vi "DataReadTxt.vi"(0 "Chemin Header":path, 5 "chemin Data":path, 9 "ScanlistIndex":i32, 11 "error in":errorcluster, 12 "VarParIndex":i32) -> (1 "Header String":string, 3 "VarPar":string, 4 "Data Preview":string[][](array[string]), 6 "X Array":dbl[](array[numeric]), 10 "Y Array":dbl[](array[numeric]), 13 "CurveName":string, 14 "enregistrement(s)":T1={"Entête"="", "Scan list"=[], "NbCourbe"=1, "IndCourbe"=0, "NomDon"=["RTêta;", "X&Y;"], "Session "=0, "Date"="", "Time"="", "VarParams"=[], "UserName"="", "ScanTableSize"=[], "VarPar list"=[], "DescKeyword"=""} caption="ScanParams", 15 "error out":errorcluster)   [LabVIEW 2019]
doc: "Ce VI lit les données contenu dans le fichier de sauvegarde automatique. Ces données correspondent aux valeurs prises lors du dernier balayage. La sauvegarde automatique est effectué après chaque acquisition."
uses:
  Interface Class/ScanParams.ctl
  Interface Class/ScanParamsOld.ctl
  Interface Class/Interface.lvclass
panel:
  out "AllData":dbl[][](array[numeric]) format="%#.16f"
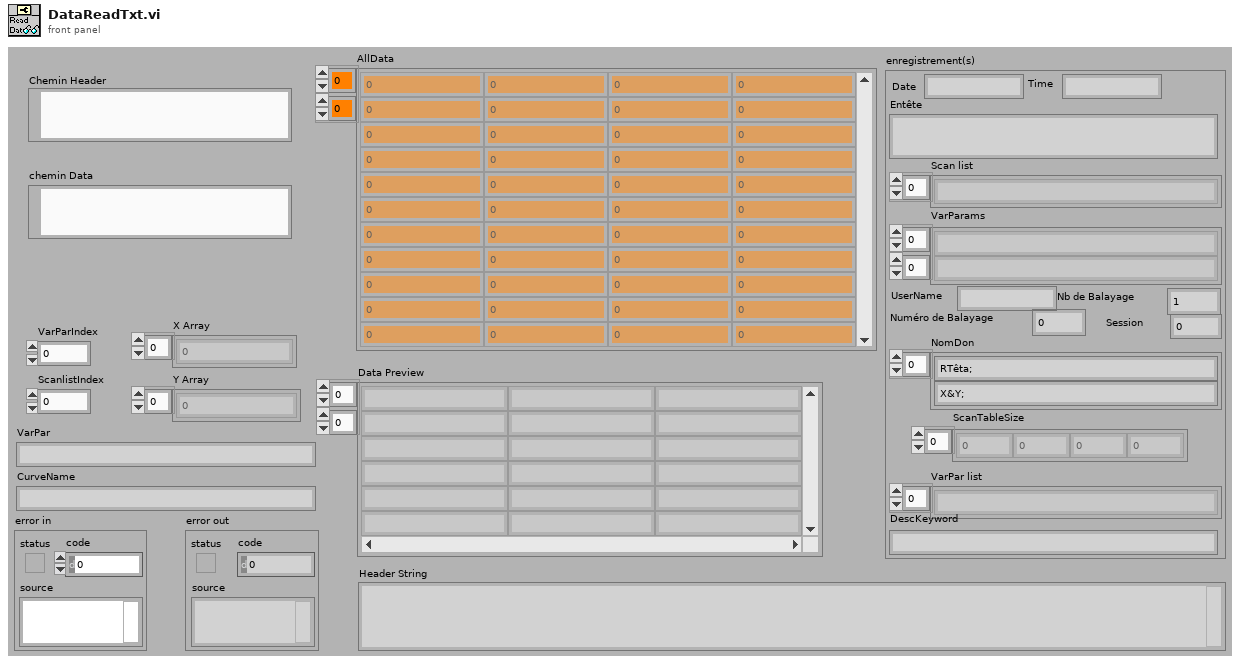
[diagram p1: front panel]
types:
  T1 = typedef "Interface.lvclass/ScanParams.ctl" = cluster{"Entête":string, "Scan list":string[], "NbCourbe":i32, "IndCourbe":i64, "NomDon":string[], "Session ":i32, "Date":string, "Time":string, "VarParams":string[][], "UserName":string, "ScanTableSize":i32[], "VarPar list":string[], "DescKeyword":string}
  T2 = typedef "Interface.lvclass/ScanParamsOld.ctl" = cluster{"Entête":string, "Scan list":string[], "NbCourbe":i32, "IndCourbe":i64, "NomDon":string[], "Session ":i32, "Date":string, "Time":string, "VarParams":string[][], "UserName":string, "ScanTableSize":i32[], "VarPar list":string[]}
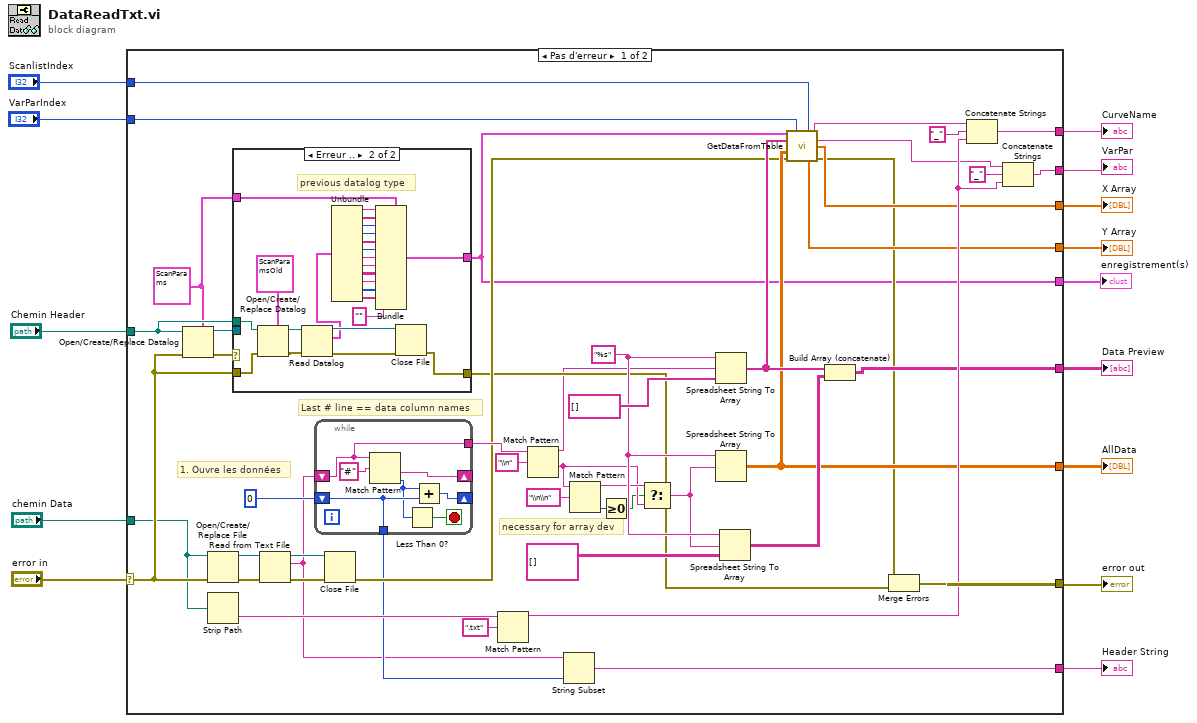
[diagram p0: block diagram]
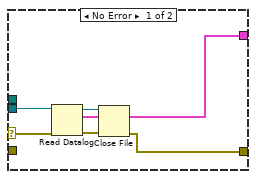
[diagram p2: hidden frame]
diagram:
  n1 = case shown="Pas d'erreur" "error in" {
    selector: "error in" -> [w31 w100]
    tunnel: "chemin Data" -> [w18 _]
    tunnel: [w33 w100] -> w14
    tunnel: [w46 _] -> w11
    tunnel: [w43 _] -> w10
    tunnel: "Chemin Header" -> [w17 _]
    tunnel: "ScanlistIndex" -> [w35 _]
    tunnel: "VarParIndex" -> [w36 _]
    tunnel: [w40 _] -> w6
    tunnel: [w39 _] -> w5
    tunnel: [w51 _] -> w4
    tunnel: [w53 _] -> w3
    tunnel: [w29 _] -> w2
    tunnel: [w15 _] -> w1
    frame No Error {
      w16 = T1 {"Entête"="", "Scan list"=[], "NbCourbe"=1, "IndCourbe"=1, "NomDon"=["RTêta;", "X&Y;"], "Session "=0, "Date"="", "Time"="", "VarParams"=[], "UserName"="", "ScanTableSize"=[], "VarPar list"=[], "DescKeyword"=""} ("ScanParams")
      w48 = "%s" ("chaîne de format")
      # "necessary for array dev"
      # "Last # line == data column names"
      # "1. Ouvre les données"
      n2 = Open/Create/Replace Datalog(5:w16, 8:w31, 11:w17) -> (0:w34:errorcluster, 3:w56:refnum<k1>)  [unwired: 3 in, 1 out]
      n3 = Open/Create/Replace File(file path (use dialog)=w18, error in=w31) -> (refnum out=w62:refnum<file>, error out=w61:errorcluster)  [unwired: 4 in, 1 out]
      n4 = Strip Path(path=w18) -> (name=w55:string)  [unwired: 1 out]
      n5 = case shown="Erreur .." w34 {
        selector: w34 -> [w65 _]
        tunnel: w56 -> [w68 _]
        tunnel: [w63 w71] -> w15
        tunnel: w17 -> [_ w87]
        tunnel: [w64 w72] -> w32
        tunnel: w31 -> [_ w70]
        tunnel: w16 -> [_ w69]
        frame No Error {
          n6 = Read Datalog(4:w65, 7:w68) -> (0:w67:errorcluster, 2:w63:T1, 3:w66:refnum<k1>)  [unwired: 1 in]
          n7 = Close File(refnum=w66, error in=w67) -> (error out=w64:errorcluster)  [unwired: 1 out]
        }
        frame Error {
          # "previous datalog type"
          n8 = Open/Create/Replace Datalog(5:T2 {"Entête"="", "Scan list"=[], "NbCourbe"=1, "IndCourbe"=1, "NomDon"=["RTêta;", "X&Y;"], "Session "=0, "Date"="", "Time"="", "VarParams"=[], "UserName"="", "ScanTableSize"=[], "VarPar list"=[]} ("ScanParams"), 8:w70, 11:w87) -> (0:w89:errorcluster, 3:w90:refnum<k1>)  [unwired: 3 in, 1 out]
          n9 = Read Datalog(4:w89, 7:w90) -> (0:w92:errorcluster, 2:w86:T2, 3:w91:refnum<k1>)  [unwired: 1 in]
          n10 = Unbundle(w86) -> ("Entête"=w85:string, "Scan list"=w84:string[], "NbCourbe"=w83:i32, "IndCourbe"=w82:i64, "NomDon"=w81:string[], "Session"=w80:i32, "Date"=w79:string, "Time"=w78:string, "VarParams"=w77:string[][], "UserName"=w76:string, "ScanTableSize"=w75:i32[], "VarPar list"=w74:string[])
          n11 = Bundle(cluster=w69, "Entête"=w85, "Scan list"=w84, "NbCourbe"=w83, "IndCourbe"=w82, "NomDon"=w81, "Session"=w80, "Date"=w79, "Time"=w78, "VarParams"=w77, "UserName"=w76, "ScanTableSize"=w75, "VarPar list"=w74, "DescKeyword"="") -> (w71:T1)
          n12 = Close File(refnum=w91, error in=w92) -> (error out=w72:errorcluster)  [unwired: 1 out]
        }
      }
      n13 = Read from Text File(file (use dialog)=w62, error in=w61) -> (refnum out=w59:refnum<file>, text=w19:string, error out=w60:errorcluster)  [unwired: 2 in, 1 out]
      n14 = while {
        shift-right: [w98] -> _
        shift-left: w19 -> [w96]
        tunnel: [w96] -> w58
        shift-right: [w93] -> _
        shift-left: 0 ("offset past match") -> [w95]
        tunnel: [w95] -> w27
        stop <- w97 stop-if-true
        n15 = Match Pattern(string=w96, regular expression="#" ("expression régulière")) -> (after substring=w98:string, offset past match=w94:i32)  [unwired: 1 in, 2 out]
        n16 = Less Than 0?(x=w94) -> (x < 0?=w97:bool)
        n17 = Add(x=w94, y=w95) -> (x+y=w93:i32)
      }
      n18 = Close File(refnum=w59, error in=w60) -> (error out=w37:errorcluster)  [unwired: 1 out]
      n19 = Match Pattern(string=w55, regular expression=".txt" ("expression régulière")) -> (before substring=w50:string)  [unwired: 1 in, 3 out]
      n20 = Match Pattern(string=w58, regular expression="\\n" ("expression régulière")) -> (before substring=w20:string, after substring=w23:string)  [unwired: 1 in, 2 out]
      n21 = String Subset(string=w19, length (rest)=w27) -> (substring=w29:string)  [unwired: 1 in]
      n22 = Match Pattern(string=w23, regular expression="\\n\\n" ("expression régulière")) -> (before substring=w25:string, offset past match=w21:i32)  [unwired: 1 in, 2 out]
      n23 = Greater Or Equal To 0?(x=w21) -> (x >= 0?=w22:bool)
      n24 = Select(t=w25, s=w22, f=w23) -> (s? t:f=w24:string)
      n25 = Spreadsheet String To Array(format string=w48, spreadsheet string=w20, array type (2D Dbl)=string[] []) -> (array=w44:string[])  [unwired: 1 in]
      n26 = Spreadsheet String To Array(format string=w48, spreadsheet string=w24) -> (array=w43:dbl[][])  [unwired: 2 in]
      n27 = Spreadsheet String To Array(format string=w48, spreadsheet string=w24, array type (2D Dbl)=string[][] []) -> (array=w47:string[][])  [unwired: 1 in]
      n28 = call "GetDataFromTable.vi"("DataRecord"=w15, "XVarParIndex"=w36, "ScanlistIndex"=w35, "FilesColName"=w44, "AllDataIn"=w43, "error in"=w37) -> ("CurveName"=w42:string, "VarPar"=w41:string, "X Array"=w39:dbl[], "Data Array"=w40:dbl[], "error out"=w38:errorcluster)  [unwired: 2 in, 3 out]
      n29 = Build Array (concatenate)(w44, w47) -> (w46:string[][])
      n30 = Merge Errors(w38, w32) -> (w33:errorcluster)
      n31 = Concatenate Strings(w42, "_" ("chaîne"), w50) -> (w53:string)
      n32 = Concatenate Strings(w41, "_" ("chaîne"), w50) -> (w51:string)
    }
    frame Error {
    }
  }
  "error out" <- w14
  "Data Preview" <- w11
  "AllData" <- w10
  "Y Array" <- w6
  "X Array" <- w5
  "VarPar" <- w4
  "CurveName" <- w3
  "Header String" <- w2
  "enregistrement(s)" <- w1
